vi "EVM high limit.vi"(11 "MCS Index":string) -> (3 "EVM High Limit":dbl=-28.0)   [LabVIEW 2012]
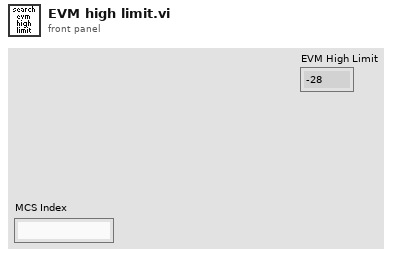
[diagram p1: front panel]
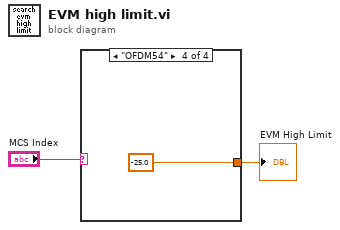
[diagram p0: block diagram]
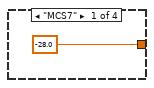
[diagram p2: hidden frame]
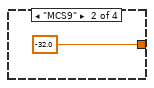
[diagram p3: hidden frame]
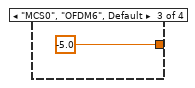
[diagram p4: hidden frame]
diagram:
  n1 = case shown="\"OFDM54\"" "MCS Index" {
    tunnel: [-28.0 -32.0 -5.0 -25.0] -> w1
    frame "MCS7" {
    }
    frame "MCS9" {
    }
    frame "MCS0", "OFDM6", Default {
    }
    frame "OFDM54" {
    }
  }
  "EVM High Limit" <- w1
